vi "RNGTEMP.vi"() -> ()   [LabVIEW 2014]
panel:
  out "XY Graph":cluster{"X":dbl, "Y":dbl}[](graph)
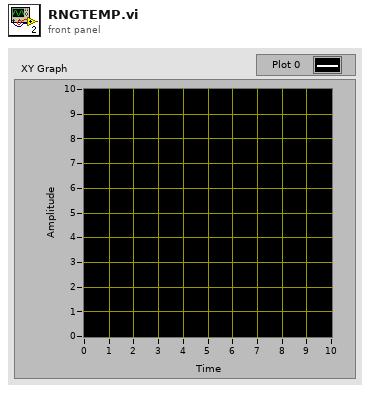
[diagram p1: front panel]
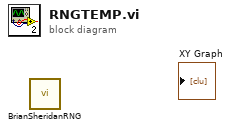
[diagram p0: block diagram]
diagram:
  n1 = call "BrianSheridanRNG.vi"() -> ()  [unwired: 2 in, 1 out]
